vi "initialise.vi"(0 "error in (no error)":errorcluster) -> (6 "Queues":T2, 7 "error out":errorcluster, 8 "configuration":T3, 9 "network streaming queues":T4, 10 "FPGA VI ref":T1)   [LabVIEW 2010]
uses:
  network_streaming_queues_cluster.ctl
  scan_specification_cluster.ctl
  config_data_cluster.ctl
  internal_queues.ctl
  line_info.ctl
  volume_with_lines.ctl
  volume_info.ctl
  kalman_result_scaled.ctl
  location3D.ctl
  spot location.ctl
  FPGA_ref.ctl
  <vilib>/userDefined/High Color/nirio_resource_hc.ctl
  <vilib>/rvi/interface/nirviOpenFPGA/nirviOpenFPGA.xnode
  FPGA Bitfiles/PCIe-7842R_main.lvbitx
  <vilib>/rvi/ClientSDK/nirviWhatTheDeviceIsDoing.ctl
  <vilib>/rvi/interface/nirviMethod/nirviMethod.xnode
  <vilib>/rvi/interface/nirviReadWriteControl/nirviReadWriteControl.xnode
  <vilib>/rvi/interface/common/niFpgaNodeNameForErrorReporting.ctl
  <vilib>/rvi/errors/niLvFpgaWhatHappensToTopLevelVI.ctl
  <vilib>/FPGAPlugInAG/PCIe-7842R/niLvFpga_Open_PCIe-7842R.vi
  <vilib>/rvi/interface/common/dynamic/niFpgaDynamicAddResources.vi
  <vilib>/Utility/error.llb/Error Cluster From Error Code.vi
  <vilib>/FPGAPlugInAG/Dynamic/niLvFpga_Reset_Dynamic.vi
  <vilib>/rvi/errors/niLvFpgaAdjustHostInterfaceError.vi
  NiFpgaLv.dll
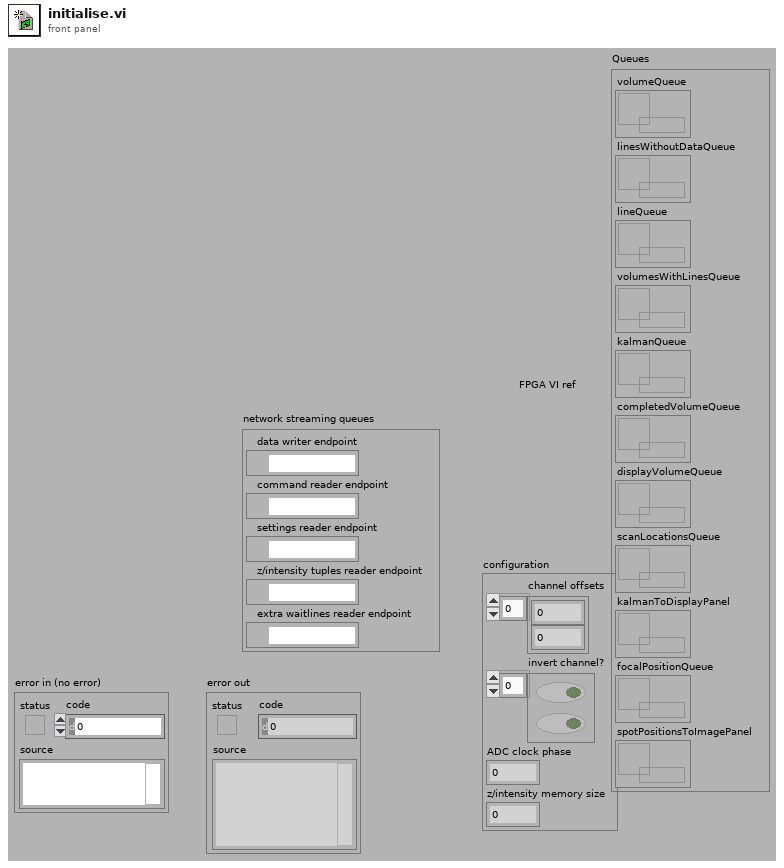
[diagram p1: front panel]
types:
  T1 = typedef "FPGA_ref.ctl" = refnum<k20>
  T2 = typedef "internal_queues.ctl" = cluster{"volumeQueue":refnum<queue>, "linesWithoutDataQueue":refnum<queue>, "lineQueue":refnum<queue>, "volumesWithLinesQueue":refnum<queue>, "kalmanQueue":refnum<queue>, "completedVolumeQueue":refnum<queue>, "displayVolumeQueue":refnum<queue>, "scanLocationsQueue":refnum<queue>, "kalmanToDisplayPanel":refnum<queue>, "focalPositionQueue":refnum<queue>, "spotPositionsToImagePanel":refnum<queue>}
  T3 = typedef "config_data_cluster.ctl" = cluster{"channel offsets":u32[], "invert channel?":bool[], "ADC clock phase":i32, "z/intensity memory size":i32}
  T4 = typedef "network_streaming_queues_cluster.ctl" = cluster{"data writer endpoint":refnum<k21>, "command reader endpoint":refnum<k21>, "settings reader endpoint":refnum<k21>, "z/intensity tuples reader endpoint":refnum<k21>, "extra waitlines reader endpoint":refnum<k21>}
  T5 = typedef "scan_specification_cluster.ctl" = cluster{"x amplitude":u16, "x resolution (pixels)":u16, "x offset fly-forward (iterations)":u16, "x offset fly-back (iterations)":u16, "y resolution (nr. of lines)":u16, "y step size":u16, "iterations per pixel":u16, "number of frames":i32, "y offset (pixels)":u16, "number of y-brake lines  (before y-fly-back)":u16, "number y-brake lines (after y-fly-back)":u16, "number of y-fly-back steps":u16, "lines per z step":u16, "number of z/intensity tuples":u16, "number of repetitions (volumes or planes)":i32, "z step size derived":u16, "choose the beginning of z scan":bool, "number of frames (settings)":i32, "FPGA trajectory?":bool, "Pockels cell voltage (bits)":i16, "Vy min(bits)":i16, "Vz min(bits)":i16}
  T6 = typedef "nirio_resource_hc.ctl" = tag
  T7 = typedef "niFpgaNodeNameForErrorReporting.ctl" = enum16{"Open FPGA VI Reference", "Read/Write Control", "Invoke Method: Abort", "Invoke Method: Acknowledge IRQ", "Invoke Method: Download", "Invoke Method: FIFO.Configure", "Invoke Method: FIFO.Read", "Invoke Method: FIFO.Start", "Invoke Method: FIFO.Stop", "Invoke Method: FIFO.Write", "Invoke Method: Reset", "Invoke Method: Run", "Invoke Method: Wait on IRQ", "Close FPGA VI Reference"}
  T8 = typedef "niLvFpgaWhatHappensToTopLevelVI.ctl" = enum16{"top level VI scripted behind XNode", "top level VI inlined behind XNode"}
  T9 = typedef "nirviWhatTheDeviceIsDoing.ctl" = enum32{"nothing", "something other than LabVIEW FPGA", "FPGA interface", "interactive", "emulation"}
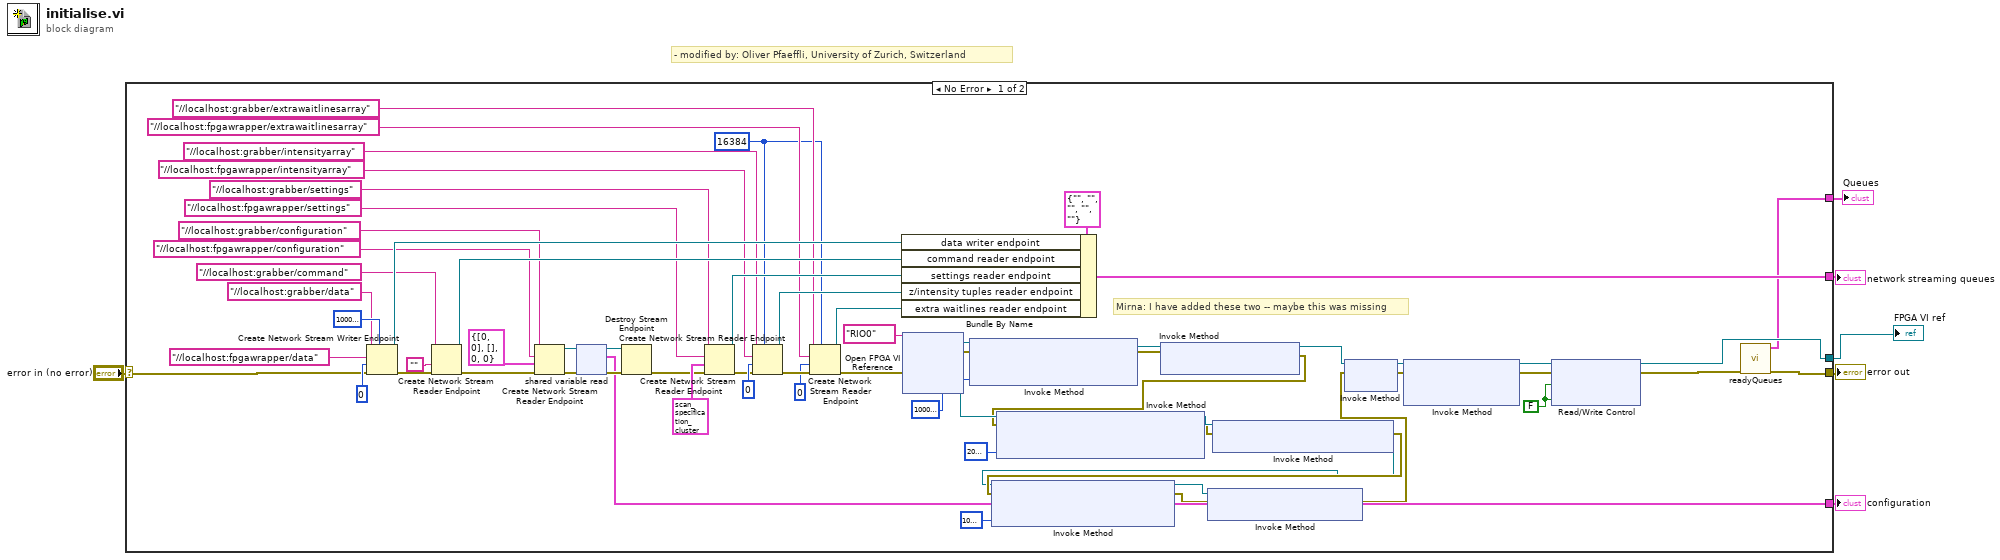
[diagram p0: block diagram]
diagram:
  # "- modified by: Oliver Pfaeffli, University of Zurich, Switzerland"
  n1 = case shown="No Error" "error in (no error)" {
    selector: "error in (no error)" -> [w47 w370]
    tunnel: [w21 w370] -> w5
    tunnel: [w65 _] -> w1
    tunnel: [w58 _] -> w4
    tunnel: [w45 _] -> w3
    tunnel: [w20 _] -> w2
    frame No Error {
      w26 = 16384 ("reader buffer size")
      w7 = FALSE ("FIFO overflow")
      # "Mirna: I have added these two -- maybe this was missing"
      n2 = Create Network Stream Writer Endpoint(7:10000000 ("writer buffer size"), 8:w47, 9:u32 0, 10:"//localhost:fpgawrapper/data" ("reader url"), 11:"//localhost:grabber/data" ("writer name")) -> (0:w55:errorcluster, 3:w59:refnum<k21>)  [unwired: 1 in]
      n3 = Create Network Stream Reader Endpoint(8:w55, 9:"", 11:"//localhost:grabber/command" ("reader name")) -> (0:w33:errorcluster, 3:w54:refnum<k21>)  [unwired: 3 in]
      n4 = Create Network Stream Reader Endpoint(8:w33, 9:T3 {"channel offsets"=[0, 0], "invert channel?"=[], "ADC clock phase"=0, "z/intensity memory size"=0} ("configuration"), 10:"//localhost:fpgawrapper/configuration" ("writer name"), 11:"//localhost:grabber/configuration" ("reader name")) -> (0:w50:errorcluster, 3:w49:refnum<k21>)  [unwired: 2 in]
      n5 = shared-variable-read(w49, w50) -> (w48:refnum<k21>, w51:errorcluster, w45:T3)  [unwired: 1 in, 1 out]
      n6 = Destroy Stream Endpoint(8:w51, 11:w48) -> (0:w35:errorcluster)
      n7 = Create Network Stream Reader Endpoint(8:w35, 9:T5 {"x amplitude"=0, "x resolution (pixels)"=0, "x offset fly-forward (iterations)"=0, "x offset fly-back (iterations)"=0, "y resolution (nr. of lines)"=0, "y step size"=0, "iterations per pixel"=0, "number of frames"=0, "y offset (pixels)"=0, "number of y-brake lines  (before y-fly-back)"=0, "number y-brake lines (after y-fly-back)"=0, "number of y-fly-back steps"=0, "lines per z step"=0, "number of z/intensity tuples"=0, "number of repetitions (volumes or planes)"=0, "z step size derived"=0, "choose the beginning of z scan"=FALSE, "number of frames (settings)"=0, "FPGA trajectory?"=FALSE, "Pockels cell voltage (bits)"=0, "Vy min(bits)"=0, "Vz min(bits)"=0} ("scan specification"), 10:"//localhost:fpgawrapper/settings" ("writer name"), 11:"//localhost:grabber/settings" ("reader name")) -> (0:w34:errorcluster, 3:w40:refnum<k21>)  [unwired: 2 in]
      n8 = Create Network Stream Reader Endpoint(7:w26, 8:w34, 9:u32 0, 10:"//localhost:fpgawrapper/intensityarray" ("writer name"), 11:"//localhost:grabber/intensityarray" ("reader name")) -> (0:w32:errorcluster, 3:w36:refnum<k21>)  [unwired: 1 in]
      n9 = Create Network Stream Reader Endpoint(7:w26, 8:w32, 9:u32 0, 10:"//localhost:fpgawrapper/extrawaitlinesarray" ("writer name"), 11:"//localhost:grabber/extrawaitlinesarray" ("reader name")) -> (0:w31:errorcluster, 3:w27:refnum<k21>)  [unwired: 1 in]
      n10 = Bundle By Name(cluster=T4 {"data writer endpoint"="", "command reader endpoint"="", "settings reader endpoint"="", "z/intensity tuples reader endpoint"="", "extra waitlines reader endpoint"=""} ("network streaming queues"), "data writer endpoint"=w59, "command reader endpoint"=w54, "settings reader endpoint"=w40, "z/intensity tuples reader endpoint"=w36, "extra waitlines reader endpoint"=w27) -> (w58:T4)
      n11 = xnode "Open FPGA VI Reference"("error in"=w31, "resource name"=T6 "RIO0") -> ("FPGA VI Reference Out"=w19:refnum<k20>, "error out"=w25:errorcluster)
      n12 = xnode "Invoke Method"("FPGA VI Reference In"=w19, "error in"=w25, "Depth"=u32 10000000) -> ("FPGA VI Reference Out"=w24:refnum<k20>, "error out"=w23:errorcluster)
      n13 = xnode "Invoke Method"("FPGA VI Reference In"=w24, "error in"=w23) -> ("FPGA VI Reference Out"=w22:refnum<k20>, "error out"=w15:errorcluster)
      n14 = xnode "Invoke Method"("FPGA VI Reference In"=w19, "error in"=w15, "Depth"=u32 2000000) -> ("FPGA VI Reference Out"=w17:refnum<k20>, "error out"=w16:errorcluster)
      n15 = xnode "Invoke Method"("FPGA VI Reference In"=w17, "error in"=w16) -> ("FPGA VI Reference Out"=w9:refnum<k20>, "error out"=w11:errorcluster)
      n16 = xnode "Invoke Method"("FPGA VI Reference In"=w9, "error in"=w11, "Depth"=u32 1000000) -> ("FPGA VI Reference Out"=w8:refnum<k20>, "error out"=w12:errorcluster)
      n17 = xnode "Invoke Method"("FPGA VI Reference In"=w8, "error in"=w12) -> ("error out"=w10:errorcluster)  [unwired: 1 out]
      n18 = xnode "Invoke Method"("FPGA VI Reference In"=w22, "error in"=w10) -> ("FPGA VI Reference Out"=w67:refnum<k20>, "error out"=w66:errorcluster)
      n19 = xnode "Invoke Method"("FPGA VI Reference In"=w67, "error in"=w66) -> ("FPGA VI Reference Out"=w69:refnum<k20>, "error out"=w68:errorcluster)  [unwired: 1 out]
      n20 = xnode "Read/Write Control"("FPGA VI Reference In"=w69, "error in"=w68, "FIFO overflow"=w7, "stop"=w7) -> ("FPGA VI Reference Out"=w65:refnum<k20>, "error out"=w46:errorcluster)
      n21 = call "readyQueues.vi"("error in (no error)"=w46) -> ("error out"=w21:errorcluster, "Queues"=w20:T2)  [unwired: 9 in]
    }
    frame Error {
    }
  }
  "error out" <- w5
  "network streaming queues" <- w4
  "configuration" <- w3
  "Queues" <- w2
  "FPGA VI ref" <- w1
